vi "Init.vi"(8 "error in (no error)":errorcluster, 11 "Mock In":refnum<class "Mock.lvclass">) -> (0 "error out":errorcluster, 3 "Mock Out":refnum<class "Mock.lvclass">)   [LabVIEW 2020, in "Mock.lvclass"]
uses:
  Mock.lvclass
  Expectation/Expectation.lvclass
  VI Call/VI Call.lvclass
  Mock.lvclass/Mock.ctl
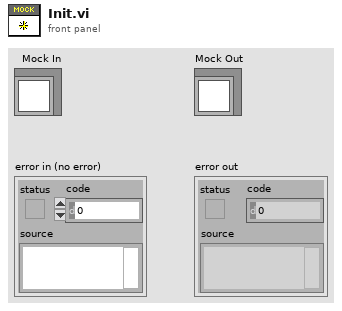
[diagram p1: front panel]
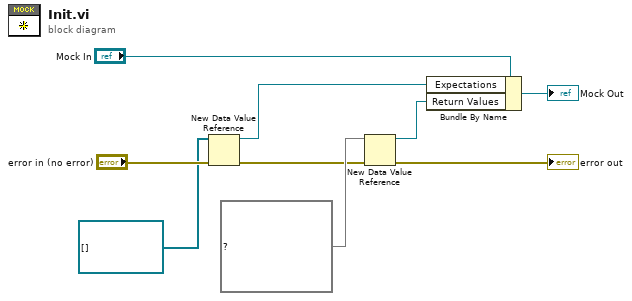
[diagram p0: block diagram]
diagram:
  n1 = New Data Value Reference(data value=refnum<class "Expectation.lvclass">[] [] ("Array"), error in="error in (no error)") -> (data value reference=w5:refnum<data-value>, error out=w2:errorcluster)
  n2 = New Data Value Reference(data value=map{string, refnum<queue>} {} ("Return Values 2"), error in=w2) -> (data value reference=w3:refnum<data-value>, error out=→"error out":errorcluster)
  n3 = Bundle By Name(cluster="Mock In", "Expectations"=w5, "Return Values"=w3) -> (→"Mock Out":refnum<class "Mock.lvclass">)
